vi "Test Smaller Hash.vi"() -> ()   [LabVIEW 2012]
panel:
  out "64-bit length":i32
  out "Hash (64 bit)":string
  out "32-bit length":i32
  in  "Lockout Date 1":timestamp format="%<%x>T"
  in  "ID":string
  out "Hash (32-bit)":string
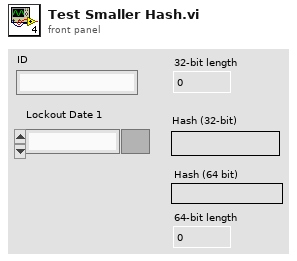
[diagram p1: front panel]
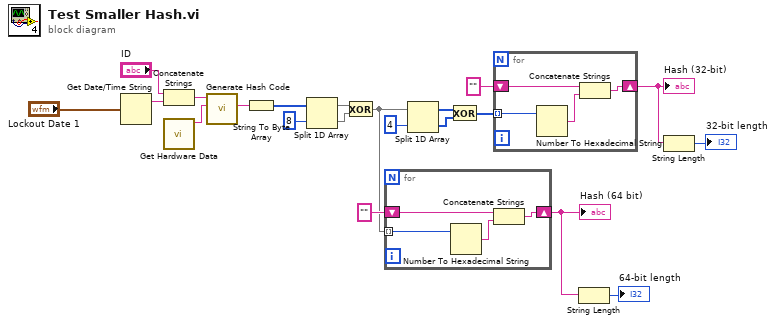
[diagram p0: block diagram]
diagram:
  n1 = Get Date/Time String(seconds (now)="Lockout Date 1") -> (date string=w21:string)  [unwired: 2 in, 1 out]
  n2 = Concatenate Strings("ID", w21) -> (w20:string)
  n3 = call "Get Hardware Data.vi"() -> ("Fingerprint"=w19:string)  [unwired: 11 in]
  n4 = call "Generate Hash Code.vi"("Fingerprint"=w19, "Product ID"=w20) -> ("Hash"=w15:string)  [unwired: 8 in, 1 out]
  n5 = String To Byte Array(string=w15) -> (unsigned byte array=w14:u8[])
  n6 = Split 1D Array(array=w14, index=8) -> (first subarray=w12:u8[], second subarray=w11:u8[])
  n7 = Exclusive Or(1:w11, 2:w12) -> (0:w3:u8[])
  n8 = for {
    tunnel: w3 -> [w25] mode=indexing
    shift-right: [w23] -> w2
    shift-left: "" -> [w22]
    n9 = Number To Hexadecimal String(2:w25) -> (0:w24:string)  [unwired: 1 in]
    n10 = Concatenate Strings(w22, w24) -> (w23:string)
  }
  "Hash (64 bit)" <- w2
  n11 = Split 1D Array(array=w3, index=4) -> (first subarray=w9:u8[], second subarray=w8:u8[])
  n12 = Exclusive Or(1:w8, 2:w9) -> (0:w7:u8[])
  n13 = for {
    tunnel: w7 -> [w29] mode=indexing
    shift-right: [w27] -> w5
    shift-left: "" -> [w26]
    n14 = Number To Hexadecimal String(2:w29) -> (0:w28:string)  [unwired: 1 in]
    n15 = Concatenate Strings(w26, w28) -> (w27:string)
  }
  "Hash (32-bit)" <- w5
  n16 = String Length(string=w2) -> (length=→"64-bit length":i32)
  n17 = String Length(string=w5) -> (length=→"32-bit length":i32)
